vi "TWM Client Cmd Get Result.vi"(4 "phase ref channel tag (none)":string, 5 "timeout [s] (10s)":dbl=10.0, 6 "qwtb maxdim (scalar)":T3 caption="Max. shown dimension (scalar)", 7 "end of packet key":string="TWM:command:EndOfPacket", 8 "error in":errorcluster, 9 "quantity names (all)":string[](array[string]), 10 "meas root path (last)":path, 11 "handle":i32) -> (0 "error out":errorcluster, 1 "result info":T1, 2 "result data":T2[][](array[typedef]), 3 "handle out":i32)   [LabVIEW 2020, in "TWM Client.lvlib"]
doc: "Write Get result command packet to TWM server. Get answer. Set reasonable timeout for the TWM processing, because it has to load, process and format the result before sending."
uses:
  TWM Client.lvlib
  TWM Client Result Max Dim.ctl
  TWM Client Quantity Record.ctl
  TWM Client Result Info.ctl
  String.vi
  1D String.vi
  I64.vi
  EXT.vi
  Get 1D String.vi
  <vilib>/Utility/error.llb/Error Cluster From Error Code.vi
  GetString.vi
  GetBoolean.vi
  Get 1D EXT.vi
  GetI64.vi
  <vilib>/ErrorRing/Error Ring.xnode
  infolib.lvlib
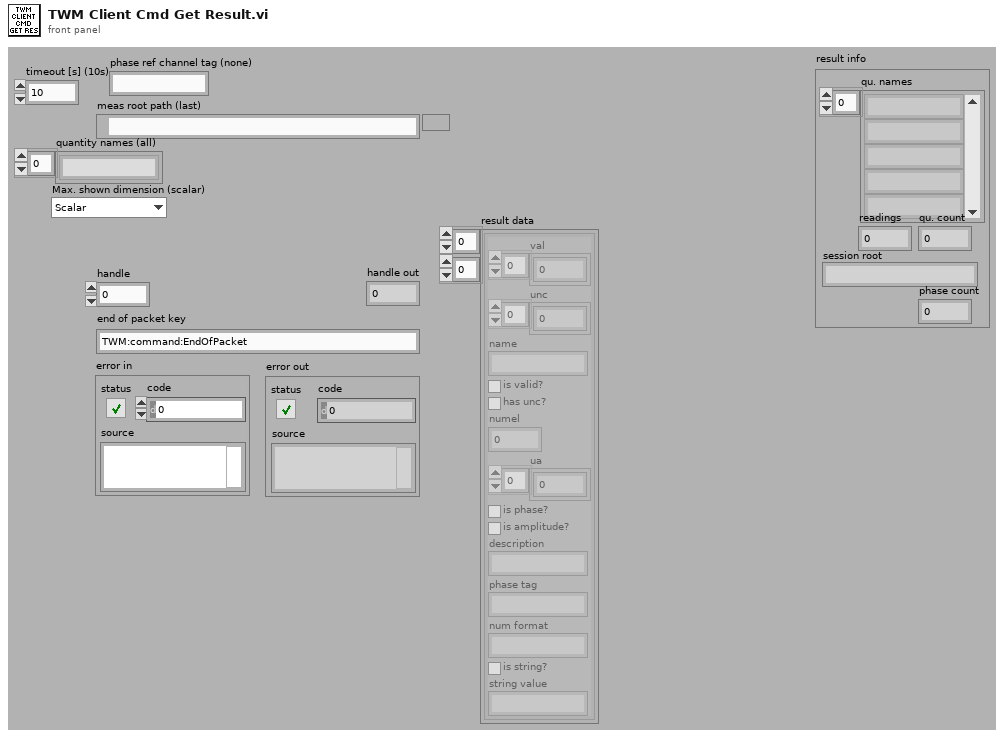
[diagram p1: front panel]
types:
  T1 = typedef "TWM Client.lvlib/TWM Client Result Info.ctl" = cluster{"qu. names":string[], "readings":i32, "qu. count":i32, "session root":string, "phase count":i32}
  T2 = typedef "TWM Client.lvlib/TWM Client Quantity Record.ctl" = cluster{"val":dbl[], "unc":dbl[], "name":string, "is valid?":bool, "has unc?":bool, "numel":i32, "ua":dbl[], "is phase?":bool, "is amplitude?":bool, "description":string, "phase tag":string, "num format":string, "is string?":bool, "string value":string}
  T3 = typedef "TWM Client.lvlib/TWM Client Result Max Dim.ctl" = enum16{"Scalar", "Vector", "Matrix"}
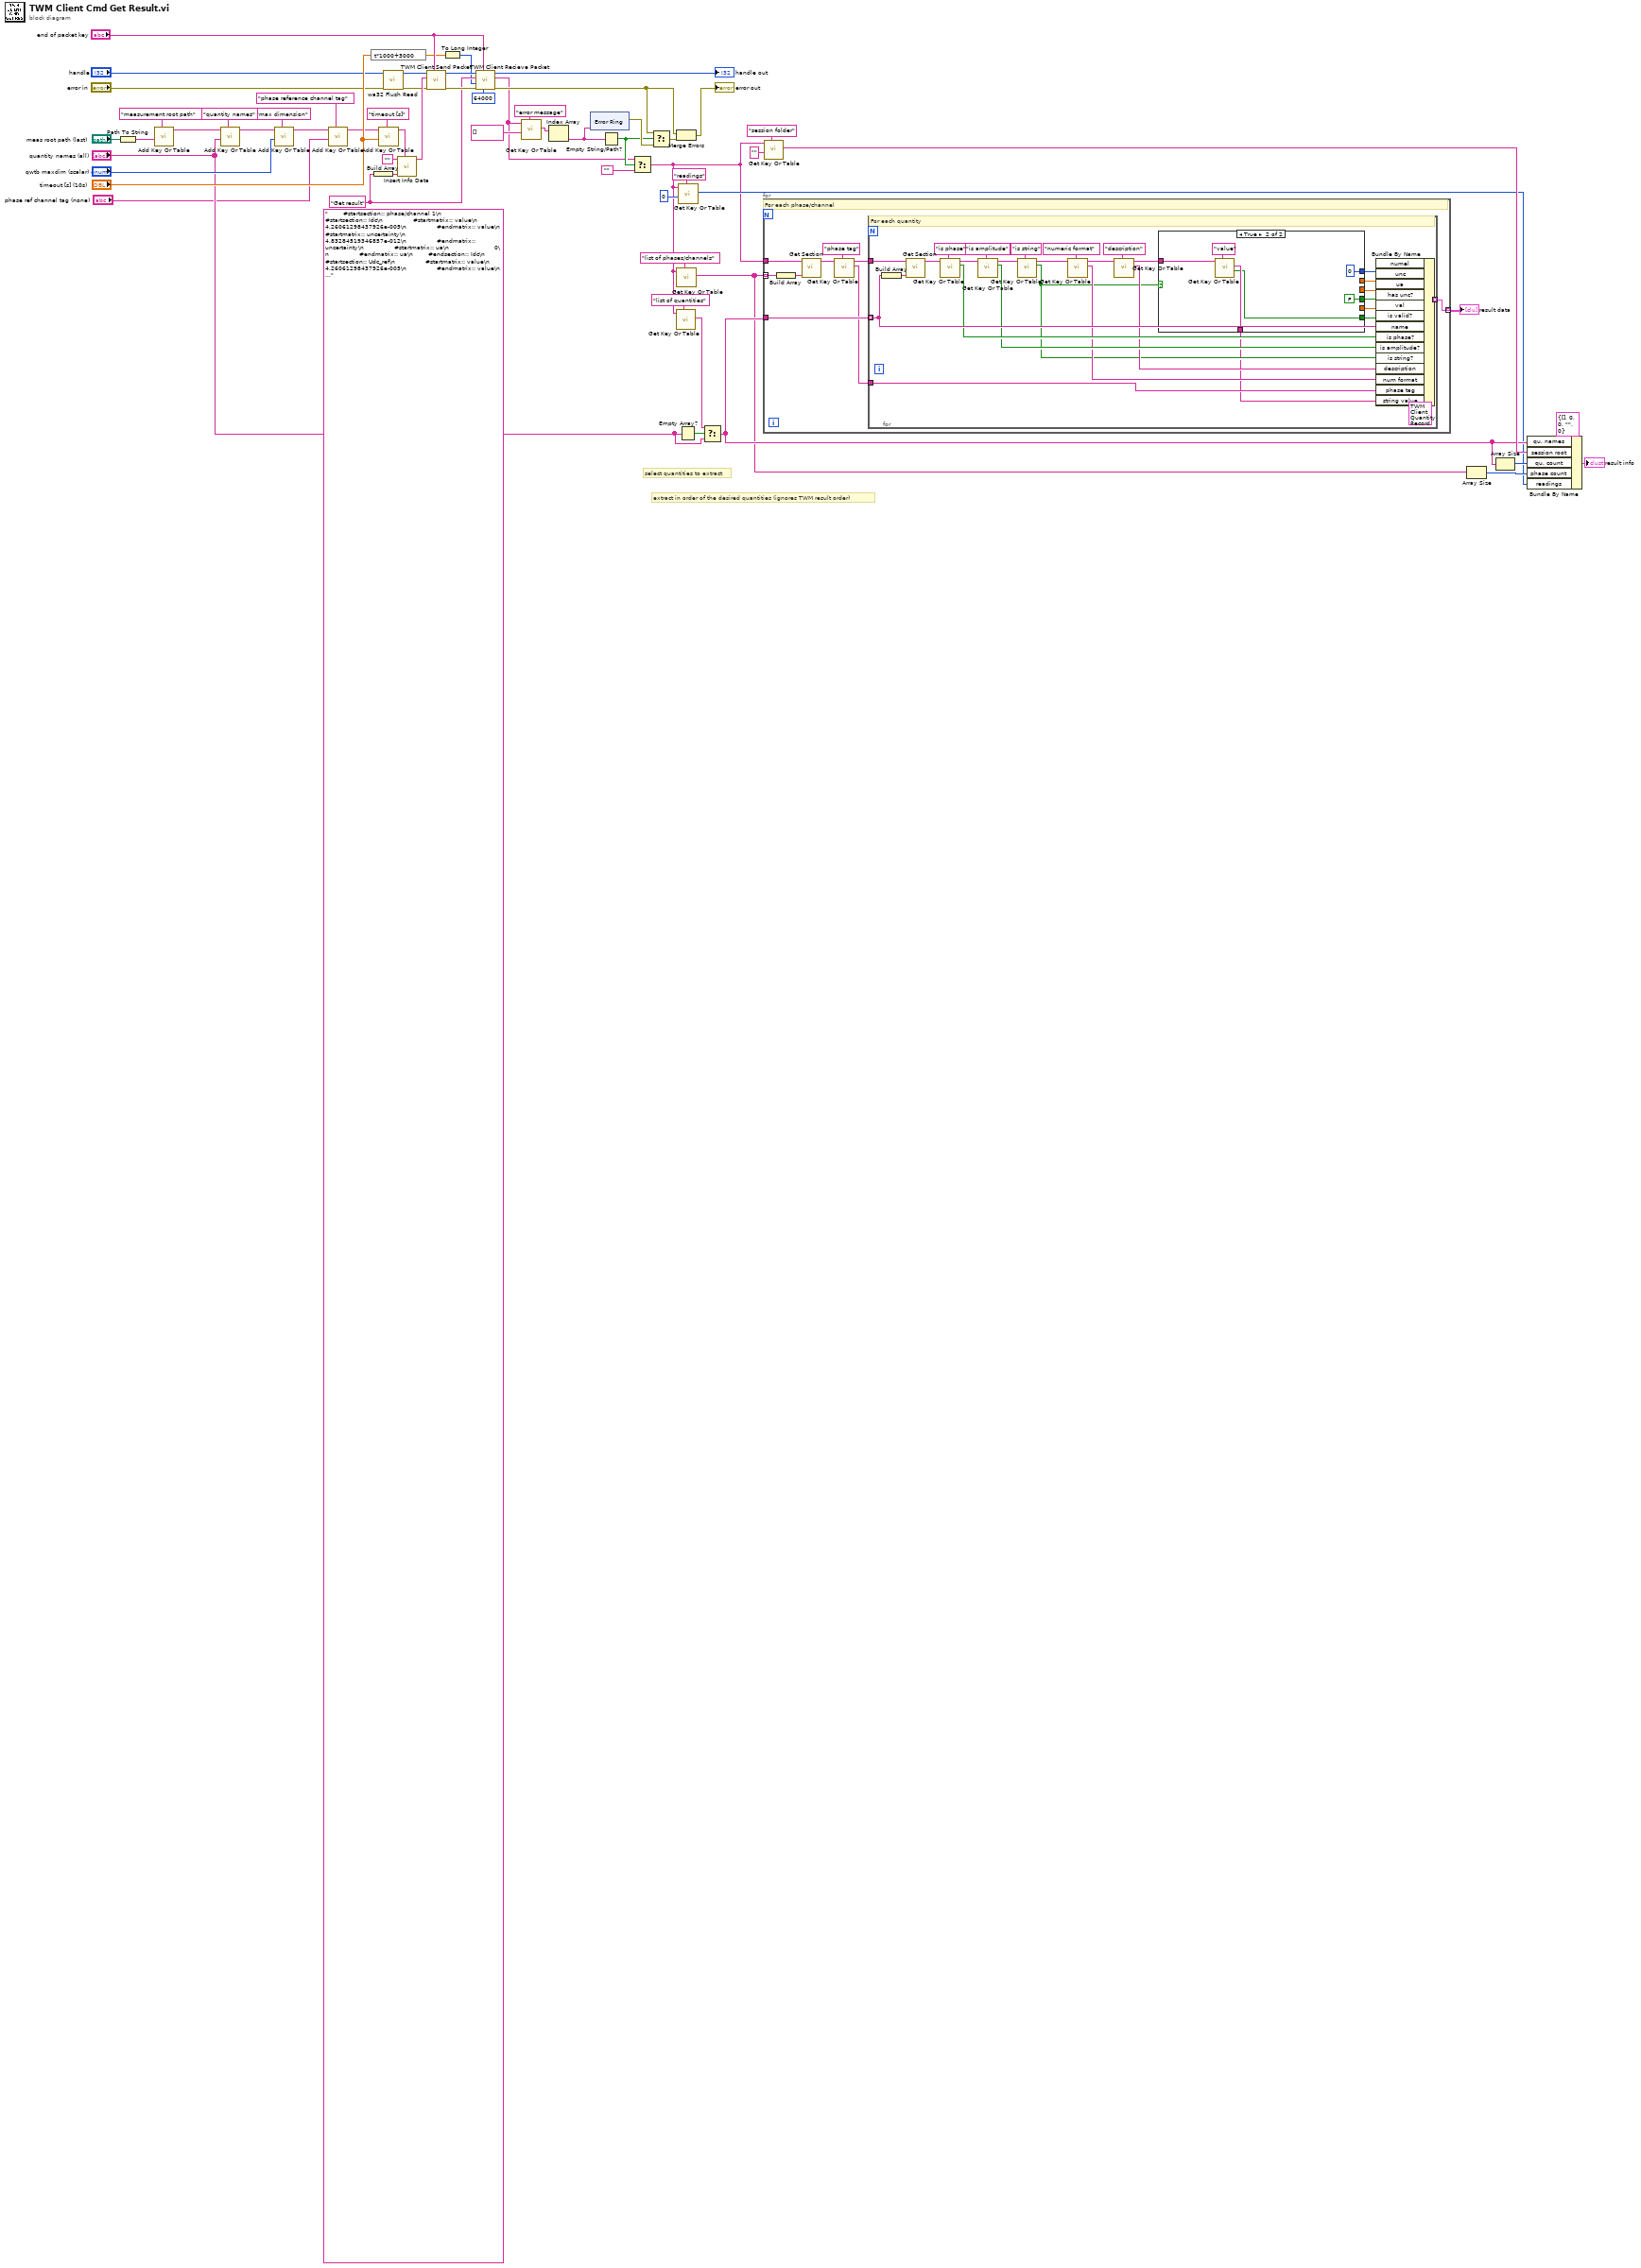
[diagram p0: block diagram]
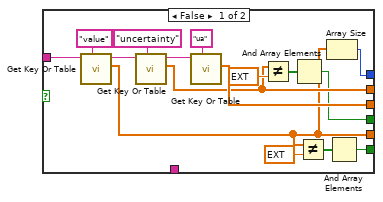
[diagram p2: hidden frame]
diagram:
  (unwired) "        #startsection:: phase/channel 1\n        #startsection:: Idc\n                #startmatrix:: value\n                        4.26061298437926e-005\n                #endmatrix:: value\n                #startmatrix:: uncertainty\n                        4.83284519346857e-012\n                #endmatrix:: uncertainty\n                #startmatrix:: ua\n                        0\n                #endmatrix:: ua\n        #endsection:: Idc\n        #startsection:: Udc_ref\n                #startmatrix:: value\n                        4.26061298437926e-005\n                #endmatrix:: value\n                #startmatrix:: uncertainty\n                        4.83284519346857e-012\n                #endmatrix:: uncertainty\n                #startmatrix:: ua\n                        0\n                #endmatrix:: ua\n        #endsection:: Udc_ref\n        #startsection:: Udc\n                #startmatrix:: value\n                        4.303281131875e-005\n                #endmatrix:: value\n                #startmatrix:: uncertainty\n                        2.41690177471195e-012\n                #endmatrix:: uncertainty\n                #startmatrix:: ua\n                        0\n                #endmatrix:: ua\n        #endsection:: Udc\n        #startsection:: Iref\n                #startmatrix:: value\n                        0.00294025760782506\n                #endmatrix:: value\n                #startmatrix:: uncertainty\n                        0\n                #endmatrix:: uncertainty\n                #startmatrix:: ua\n                        0\n                #endmatrix:: ua\n        #endsection:: Iref\n        #startsection:: Udut\n                #startmatrix:: value\n                        0.00147042022143473\n                #endmatrix:: value\n                #startmatrix:: uncertainty\n                        0\n                #endmatrix:: uncertainty\n                #startmatrix:: ua\n                        0\n                #endmatrix:: ua\n        #endsection:: Udut\n        #startsection:: mjr\n                #startmatrix:: value\n                        0.500099112921746\n                #endmatrix:: value\n                #startmatrix:: uncertainty\n                        5.99134834829246e-013\n                #endmatrix:: uncertainty\n                #startmatrix:: ua\n                        0\n                #endmatrix:: ua\n        #endsection:: mjr\n        #startsection:: mnr\n                #startmatrix:: value\n                        0.000442017712722453\n                #endmatrix:: value\n                #startmatrix:: uncertainty\n                        4.95306403476288e-010\n                #endmatrix:: uncertainty\n                #startmatrix:: ua\n                        0\n                #endmatrix:: ua\n        #endsection:: mnr\n        #startsection:: mjr_name\n                #startmatrix:: value\n                        90; 32; 91; 79; 104; 109; 93\n                #endmatrix:: value\n                #startmatrix:: uncertainty\n                        0; 0; 0; 0; 0; 0; 0\n                #endmatrix:: uncertainty\n                #startmatrix:: ua\n                        0; 0; 0; 0; 0; 0; 0\n                #endmatrix:: ua\n        #endsection:: mjr_name\n        #startsection:: mnr_name\n                #startmatrix:: value\n                        112; 104; 105; 114; 32; 91; 114; 97; 100; 93\n                #endmatrix:: value\n                #startmatrix:: uncertainty\n                        0; 0; 0; 0; 0; 0; 0; 0; 0; 0\n                #endmatrix:: uncertainty\n                #startmatrix:: ua\n                        0; 0; 0; 0; 0; 0; 0; 0; 0; 0\n                #endmatrix:: ua\n        #endsection:: mnr_name\n#endsection:: phase/channel 1\n#startsection:: phase/channel 2\n        #startsection:: Idc\n                #startmatrix:: value\n                        8.61439306713361e-005\n                #endmatrix:: value\n                #startmatrix:: uncertainty\n                        4.8322382386777e-012\n                #endmatrix:: uncertainty\n                #startmatrix:: ua\n                        0\n                #endmatrix:: ua\n        #endsection:: Idc\n        #startsection:: Udc_ref\n                #startmatrix:: value\n                        8.61439306713361e-005\n                #endmatrix:: value\n                #startmatrix:: uncertainty\n                        4.8322382386777e-012\n                #endmatrix:: uncertainty\n                #startmatrix:: ua\n                        0\n                #endmatrix:: ua\n        #endsection:: Udc_ref\n        #startsection:: Udc\n                #startmatrix:: value\n                        8.82410956791666e-005\n                #endmatrix:: value\n                #startmatrix:: uncertainty\n                        2.41777822239762e-012\n                #endmatrix:: uncertainty\n                #startmatrix:: ua\n                        0\n                #endmatrix:: ua\n        #endsection:: Udc\n        #startsection:: Iref\n                #startmatrix:: value\n                        0.00293988834221466\n                #endmatrix:: value\n                #startmatrix:: uncertainty\n                        0\n                #endmatrix:: uncertainty\n                #startmatrix:: ua\n                        0\n                #endmatrix:: ua\n        #endsection:: Iref\n        #startsection:: Udut\n                #startmatrix:: value\n                        0.00147095344403826\n                #endmatrix:: value\n                #startmatrix:: uncertainty\n                        0\n                #endmatrix:: uncertainty\n                #startmatrix:: ua\n                        0\n                #endmatrix:: ua\n        #endsection:: Udut\n        #startsection:: mjr\n                #startmatrix:: value\n                        0.500343303150816\n                #endmatrix:: value\n                #startmatrix:: uncertainty\n                        5.89993720299394e-013\n                #endmatrix:: uncertainty\n                #startmatrix:: ua\n                        0\n                #endmatrix:: ua\n        #endsection:: mjr\n        #startsection:: mnr\n                #startmatrix:: value\n                        5.93300718243483e-005\n                #endmatrix:: value\n                #startmatrix:: uncertainty\n                        5.01579424858811e-010\n                #endmatrix:: uncertainty\n                #startmatrix:: ua\n                        0\n                #endmatrix:: ua\n        #endsection:: mnr\n        #startsection:: mjr_name\n                #startmatrix:: value\n                        90; 32; 91; 79; 104; 109; 93\n                #endmatrix:: value\n                #startmatrix:: uncertainty\n                        0; 0; 0; 0; 0; 0; 0\n                #endmatrix:: uncertainty\n                #startmatrix:: ua\n                        0; 0; 0; 0; 0; 0; 0\n                #endmatrix:: ua\n        #endsection:: mjr_name\n        #startsection:: mnr_name\n                #startmatrix:: value\n                        112; 104; 105; 114; 32; 91; 114; 97; 100; 93\n                #endmatrix:: value\n                #startmatrix:: uncertainty\n                        0; 0; 0; 0; 0; 0; 0; 0; 0; 0\n                #endmatrix:: uncertainty\n                #startmatrix:: ua\n                        0; 0; 0; 0; 0; 0; 0; 0; 0; 0\n                #endmatrix:: ua\n        #endsection:: mnr_name\n#endsection:: phase/channel 2\nphases/channels count:: 2\n#startmatrix:: list of phases/channels\n        phase/channel 1\n        phase/channel 2\n#endmatrix:: list of phases/channels\n#startmatrix:: list of quantities\n        Idc\n        Udc_ref\n        Udc\n        Iref\n        Udut\n        mjr\n        mnr\n        mjr_name\n        mnr_name\n#endmatrix:: list of quantities\nreadings:: 1\nsession folder:: E:\\work\\twm\\openz\\test_shunt" ("t")
  w43 = "Get result" ("key string")
  # "extract in order of the desired quantities (ignores TWM result order)"
  # "select quantities to extract"
  n1 = Path To String(path="meas root path (last)") -> (string=w51:string)
  n2 = call-poly "Add Key Or Table.vi"("key description"="measurement root path", "string"=w51) -> ("info data out"=w54:string)  [unwired: 8 in, 1 out]
  n3 = call-poly "Add Key Or Table.vi"("key description"="quantity names", "string"="quantity names (all)", "info data"=w54) -> ("info data out"=w49:string)  [unwired: 7 in, 1 out]
  n4 = call-poly "Add Key Or Table.vi"("key description"="max dimension", "numeric"="qwtb maxdim (scalar)", "info data"=w49) -> ("info data out"=w25:string)  [unwired: 7 in, 1 out]
  n5 = call-poly "Add Key Or Table.vi"("key description"="phase reference channel tag", "string"="phase ref channel tag (none)", "info data"=w25) -> ("info data out"=w24:string)  [unwired: 7 in, 1 out]
  n6 = expression code="t*1000+3000"("timeout [s] (10s)") -> (w38:dbl)
  n7 = Build Array(w43) -> (w44:string[])
  n8 = call-poly "Add Key Or Table.vi"("key description"="timeout [s]", "numeric"="timeout [s] (10s)", "info data"=w24) -> ("info data out"=w45:string)  [unwired: 7 in, 1 out]
  n9 = call "wa32 Flush Read.vi"("error in"="error in", "handle"="handle") -> ("error out"=w2:errorcluster, "handle out"=w1:i32)  [unwired: 7 in, 1 out]
  n10 = call "Insert Info Data.vi"("info data to insert"=w45, "sections"=w44, "info data"="") -> ("info data out"=w42:string)  [unwired: 7 in, 1 out]
  n11 = call "TWM Client Send Packet.vi"("end of packet key"="end of packet key", "error in"=w2, "command string"=w42, "handle"=w1) -> ("error out"=w59:errorcluster, "handle out"=w57:i32)  [unwired: 6 in]
  n12 = To Long Integer(number=w38) -> (32bit integer=w37:i32)
  n13 = call "TWM Client Recieve Packet.vi"("max message length (1024)"=64000, "end of packet key"="end of packet key", "error in"=w59, "timeout [ms] (5000 ms)"=w37, "message header (empty)"=w43, "handle in"=w57) -> ("error out"=w34:errorcluster, "message data"=w6:string, "handle out"=→"handle out":i32)  [unwired: 3 in]
  n14 = call-poly "Get Key Or Table.vi"("key description"="error message", "string"=string[] [], "info data"=w6) -> ("value"=w35:string[])  [unwired: 5 in, 3 out]
  n15 = Index Array(array=w35) -> (element=w7:string)  [unwired: 1 in]
  n16 = xnode "Error Ring"("parameter 0"=w7) -> ("error out"=w33:errorcluster)
  n17 = Empty String/Path?(string/path=w7) -> (empty?=w32:bool)
  n18 = Select(t=w6, s=w32, f="") -> (s? t:f=w5:string)
  n19 = Select(t=w34, s=w32, f=w33) -> (s? t:f=w41:errorcluster)
  n20 = call-poly "Get Key Or Table.vi"("key description"="list of quantities", "info data"=w5) -> ("value"=w26:string[])  [unwired: 6 in, 3 out]
  n21 = Merge Errors(w34, w41) -> (→"error out":errorcluster)
  n22 = call-poly "Get Key Or Table.vi"("key description"="list of phases/channels", "info data"=w5) -> ("value"=w10:string[])  [unwired: 6 in, 3 out]
  n23 = call-poly "Get Key Or Table.vi"("key description"="readings", "numeric"=i64 0, "info data"=w5) -> ("value"=w9:i64)  [unwired: 5 in, 3 out]
  n24 = Empty Array?(array="quantity names (all)") -> (empty?=w28:bool)
  n25 = Select(t=w26, s=w28, f="quantity names (all)") -> (s? t:f=w12:string[])
  n26 = for {
    tunnel: w10 -> [w68] mode=indexing
    tunnel: w5 -> [w69]
    tunnel: w12 -> [w66]
    tunnel: [w67] -> w29 mode=indexing
    # "For each phase/channel"
    n27 = Build Array(w68) -> (w65:string[])
    n28 = call "Get Section.vi"("sections"=w65, "info data"=w69) -> ("section part"=w63:string)  [unwired: 7 in, 2 out]
    n29 = call-poly "Get Key Or Table.vi"("key description"="phase tag", "info data"=w63) -> ("value"=w61:string, "info data out"=w62:string)  [unwired: 6 in, 2 out]
    n30 = for {
      tunnel: w62 -> [w98]
      tunnel: [w96] -> w67 mode=indexing
      tunnel: w66 -> [w95] mode=indexing
      tunnel: w61 -> [w81]
      # "For each quantity"
      n31 = Build Array(w95) -> (w94:string[])
      n32 = call "Get Section.vi"("sections"=w94, "info data"=w98) -> ("section part"=w92:string)  [unwired: 7 in, 2 out]
      n33 = call-poly "Get Key Or Table.vi"("key description"="is phase", "info data"=w92) -> ("value"=w85:bool, "info data out"=w91:string)  [unwired: 6 in, 2 out]
      n34 = call-poly "Get Key Or Table.vi"("key description"="is amplitude", "info data"=w91) -> ("value"=w84:bool, "info data out"=w79:string)  [unwired: 6 in, 2 out]
      n35 = call-poly "Get Key Or Table.vi"("key description"="is string", "info data"=w79) -> ("value"=w77:bool, "info data out"=w78:string)  [unwired: 6 in, 2 out]
      n36 = call-poly "Get Key Or Table.vi"("key description"="numeric format", "info data"=w78) -> ("value"=w83:string, "info data out"=w87:string)  [unwired: 6 in, 2 out]
      n37 = call-poly "Get Key Or Table.vi"("key description"="description", "info data"=w87) -> ("value"=w82:string, "info data out"=w86:string)  [unwired: 6 in, 2 out]
      n38 = case shown="True" w77 {
        tunnel: [w104 _] -> w73
        tunnel: [w109 _] -> w74
        tunnel: w86 -> [w108 w119]
        tunnel: [w99 _] -> w75
        tunnel: [_ w118] -> w76
        tunnel: [w107 0] -> w72
        tunnel: [w103 FALSE] -> w71
        tunnel: [w100 w115] -> w70
        frame False {
          n39 = call-poly "Get Key Or Table.vi"("key description"="value", "info data"=w108) -> ("value"=w99:ext[], "info data out"=w112:string)  [unwired: 6 in, 2 out]
          n40 = call-poly "Get Key Or Table.vi"("key description"="uncertainty", "info data"=w112) -> ("value"=w104:ext[], "info data out"=w110:string)  [unwired: 6 in, 2 out]
          n41 = call-poly "Get Key Or Table.vi"("key description"="ua", "info data"=w110) -> ("value"=w109:ext[])  [unwired: 6 in, 3 out]
          n42 = Not Equal?(x=w104, y=ext nan) -> (x != y?=w106:bool[])
          n43 = And Array Elements(Boolean array=w106) -> (logical AND=w103:bool)
          n44 = Not Equal?(x=w99, y=ext nan) -> (x != y?=w102:bool[])
          n45 = Array Size(array=w99) -> (size(s)=w107:i32)
          n46 = And Array Elements(Boolean array=w102) -> (logical AND=w100:bool)
        }
        frame True {
          n47 = call-poly "Get Key Or Table.vi"("key description"="value", "info data"=w119) -> ("key found?"=w115:bool, "value"=w118:string)  [unwired: 6 in, 2 out]
        }
      }
      n48 = Bundle By Name(cluster=T2 {"val"=[], "unc"=[], "name"="", "is valid?"=FALSE, "has unc?"=FALSE, "numel"=0, "ua"=[], "is phase?"=FALSE, "is amplitude?"=FALSE, "description"="", "phase tag"="", "num format"="", "is string?"=FALSE, "string value"=""} ("quantity"), "numel"=w72, "unc"=w73, "ua"=w74, "has unc?"=w71, "val"=w75, "is valid?"=w70, "name"=w95, "is phase?"=w85, "is amplitude?"=w84, "is string?"=w77, "description"=w82, "num format"=w83, "phase tag"=w81, "string value"=w76) -> (w96:T2)
    }
  }
  "result data" <- w29
  n49 = call-poly "Get Key Or Table.vi"("key description"="session folder", "string"="", "info data"=w5) -> ("value"=w14:string)  [unwired: 5 in, 3 out]
  n50 = Array Size(array=w10) -> (size(s)=w11:i32)
  n51 = Array Size(array=w12) -> (size(s)=w13:i32)
  n52 = Bundle By Name(cluster=T1 {"qu. names"=[], "readings"=0, "qu. count"=0, "session root"="", "phase count"=0} ("result info"), "qu. names"=w12, "session root"=w14, "qu. count"=w13, "phase count"=w11, "readings"=w9) -> (→"result info":T1)
